vi "Enable ARB Custom Digital Modulation.vi"(8 "error in (no error)":errorcluster, 10 "Enable ARB Custom Digital Modulation (F: Disable)":bool, 11 "VISA resource name":refnum<visa-resource-name>) -> (0 "error out":errorcluster, 3 "VISA resource name out":refnum<visa-resource-name>)   [LabVIEW 2018, in "Agilent PSG MXG Series.lvlib"]
doc: "Enables or disables the ARB custom digital modulation capability.\n\n<b>Note:</b>\nIt is applicable for N5172B/82B with <b>Option 431</b> only."
uses:
  Agilent PSG MXG Series.lvlib
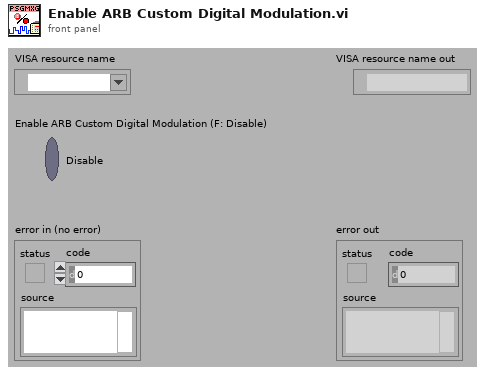
[diagram p1: front panel]
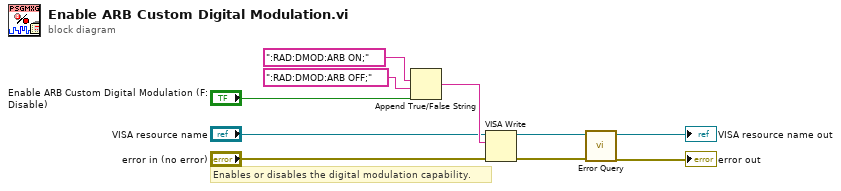
[diagram p0: block diagram]
diagram:
  # "Enables or disables the digital modulation capability."
  n1 = Append True/False String(1:"Enable ARB Custom Digital Modulation (F: Disable)", 2:":RAD:DMOD:ARB OFF;", 3:":RAD:DMOD:ARB ON;") -> (0:w7:string)  [unwired: 1 in]
  n2 = VISA Write(VISA resource name="VISA resource name", write buffer=w7, error in (no error)="error in (no error)") -> (VISA resource name out=w4:refnum<visa-resource-name>, error out=w3:errorcluster)  [unwired: 1 out]
  n3 = call "Error Query.vi"("error in (no error)"=w3, "VISA resource name"=w4) -> ("error out"=→"error out":errorcluster, "VISA resource name out"=→"VISA resource name out":refnum<visa-resource-name>)  [unwired: 6 in, 2 out]
